vi "act_DriveQuadTalonSrx.vi"(8 "error in":errorcluster, 9 "Robot Mode":T1, 11 "QuadTalonSRXDriveRef":T2={"LeftMasterDriveRef"={"DeviceStatus"={"status"=FALSE, "code"=0, "source"=""}, "Type"=enum."PWM", "PWM"={"PWM Channel"=enum."Invalid", "DeadBand"={"Name"="", "maxPositivePwm"=0, "minPositivePwm"=0, "centerPwm"=0, "maxNegativePwm"=0, "minNegativePwm"=0, "angularRange"=0}}, "CAN"={"Device Number"=0, "SetOutput VI Ref"=variant(refnum<vi> refnum), "GetOutput VI Ref"=variant(refnum<vi> refnum), "Enable VI Ref"=variant(refnum<vi> refnum), "Disable VI Ref"=variant(refnum<vi> refnum), "Data"=variant}, "Invert"=FALSE, "DIO PWM"={"PWM \"Enable\" Channel"=enum."Invalid", "DIOChannel"=enum."Invalid", "PWM Rate"=0.0}}, "RightMasterDriveRef"={"DeviceStatus"={"status"=FALSE, "code"=0, "source"=""}, "Type"=enum."PWM", "PWM"={"PWM Channel"=enum."Invalid", "DeadBand"={"Name"="", "maxPositivePwm"=0, "minPositivePwm"=0, "centerPwm"=0, "maxNegativePwm"=0, "minNegativePwm"=0, "angularRange"=0}}, "CAN"={"Device Number"=0, "SetOutput VI Ref"=variant(refnum<vi> refnum), "GetOutput VI Ref"=variant(refnum<vi> refnum), "Enable VI Ref"=variant(refnum<vi> refnum), "Disable VI Ref"=variant(refnum<vi> refnum), "Data"=variant}, "Invert"=FALSE, "DIO PWM"={"PWM \"Enable\" Channel"=enum."Invalid", "DIOChannel"=enum."Invalid", "PWM Rate"=0.0}}}) -> (0 "error out":errorcluster)   [LabVIEW 2019, in "DriveQuadTalonSRX_Motor.lvlib"]
doc: "This VI is called for each TeleOp packet received from the DS where the robot is not disabled. It is often used to read from the joysticks and update I/O or to update setpoints for timed control loops. It should complete and return within 20 milliseconds or it may miss DS packets."
uses:
  DriveQuadTalonSRX_Motor.lvlib
  <vilib>/Rock Robotics/WPI/ThirdParty/Phoenix-LabVIEW/Motor Controller/Controls/CTRE_Phoenix_MotorControl_ControlMode.ctl
  globals_DriveQuadTalonSRX.vi
  <vilib>/Rock Robotics/SystemInterfaces/DIO/FPGA_DIOPWMChannel.ctl
  <vilib>/Rock Robotics/WPI/PWM/WPI_PWMDeadband.ctl
  <vilib>/Rock Robotics/WPI/MotorControl/WPI_MotorControlType.ctl
  <vilib>/Rock Robotics/SystemInterfaces/DIO/FPGA_DIOChannel.ctl
  <vilib>/Rock Robotics/WPI/MotorControl/WPI_MotorControlDeviceRef.ctl
  ctrlRef_DriveQuadTalon.ctl
  <vilib>/Rock Robotics/WPI/DriverStation/WPI_DriverStationRobotMode2.ctl
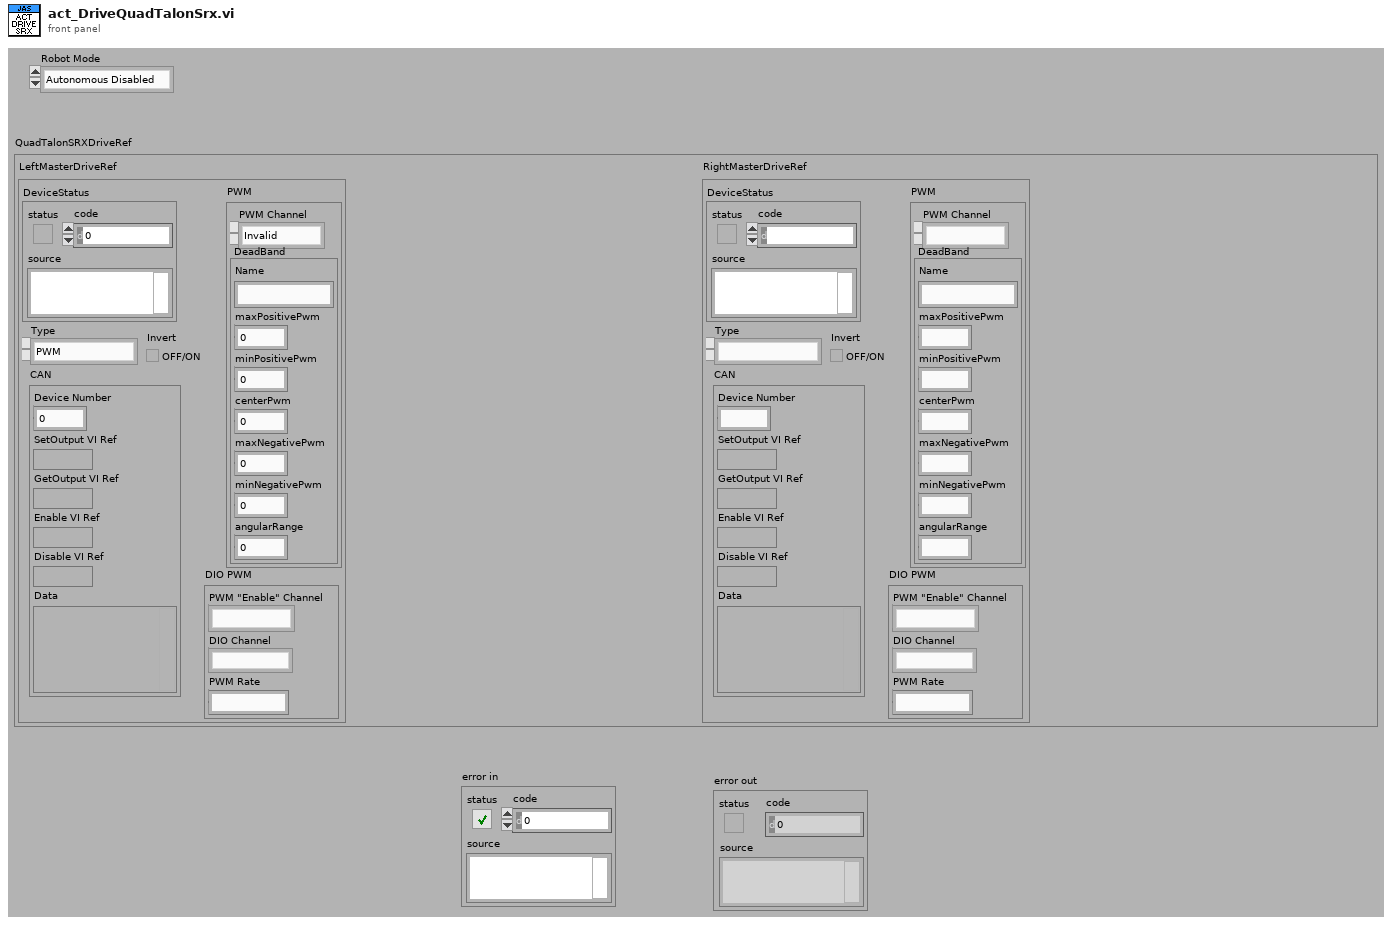
[diagram p1: front panel]
types:
  T1 = typedef "WPI_DriverStationRobotMode2.ctl" = enum16{"Autonomous Disabled", "Autonomous Enabled", "Teleop Disabled", "Teleop Enabled", "Disconnected", "Finish", "Test Disabled", "Test Enabled", "Emergency Stopped"}
  T2 = typedef "DriveQuadTalonSRX_Motor.lvlib/ctrlRef_DriveQuadTalon.ctl" = cluster{"LeftMasterDriveRef":T3, "RightMasterDriveRef":T3}
  T3 = typedef "WPI_MotorControlDeviceRef.ctl" = cluster{"DeviceStatus":errorcluster, "Type":T4, "PWM":cluster{"PWM Channel":T5, "DeadBand":T6}, "CAN":cluster{"Device Number":u8, "SetOutput VI Ref":variant, "GetOutput VI Ref":variant, "Enable VI Ref":variant, "Disable VI Ref":variant, "Data":variant}, "Invert":bool, "DIO PWM":cluster{"PWM \"Enable\" Channel":T5, "DIOChannel":T7, "PWM Rate":dbl}}
  T4 = typedef "WPI_MotorControlType.ctl" = enum16{"PWM", "CAN", "DIO PWM"}
  T5 = typedef "FPGA_DIOPWMChannel.ctl" = enum8{"PWM 0", "PWM 1", "PWM 2", "PWM 3", "PWM 4", "PWM 5", "PWM 6", "PWM 7", "PWM 8", "PWM 9", "PWM MXP 0", "PWM MXP 1", "PWM MXP 2", "PWM MXP 3", "PWM MXP 4", "PWM MXP 5", "PWM MXP 6", "PWM MXP 7", "PWM MXP 8", "PWM MXP 9", "Invalid"}
  T6 = typedef "WPI_PWMDeadband.ctl" = cluster{"Name":string, "maxPositivePwm":i32, "minPositivePwm":i32, "centerPwm":i32, "maxNegativePwm":i32, "minNegativePwm":i32, "angularRange":u16}
  T7 = typedef "FPGA_DIOChannel.ctl" = enum8{"DIO 0", "DIO 1", "DIO 2", "DIO 3", "DIO 4", "DIO 5", "DIO 6", "DIO 7", "DIO 8", "DIO 9", "DIO MXP 0", "DIO MXP 1", "DIO MXP 2", "DIO MXP 3", "DIO MXP 4", "DIO MXP 5", "DIO MXP 6", "DIO MXP 7", "DIO MXP 8", "DIO MXP 9", "DIO MXP 10", "DIO MXP 11", "DIO MXP 12", "DIO MXP 13", "DIO MXP 14", "DIO MXP 15", "SPI Port CS1", "SPI Port CS2", "SPI Port CS3", "SPI Port MISO", "SPI Port MOSI", "Invalid"}
  T8 = typedef "CTRE_Phoenix_MotorControl_ControlMode.ctl" = u16
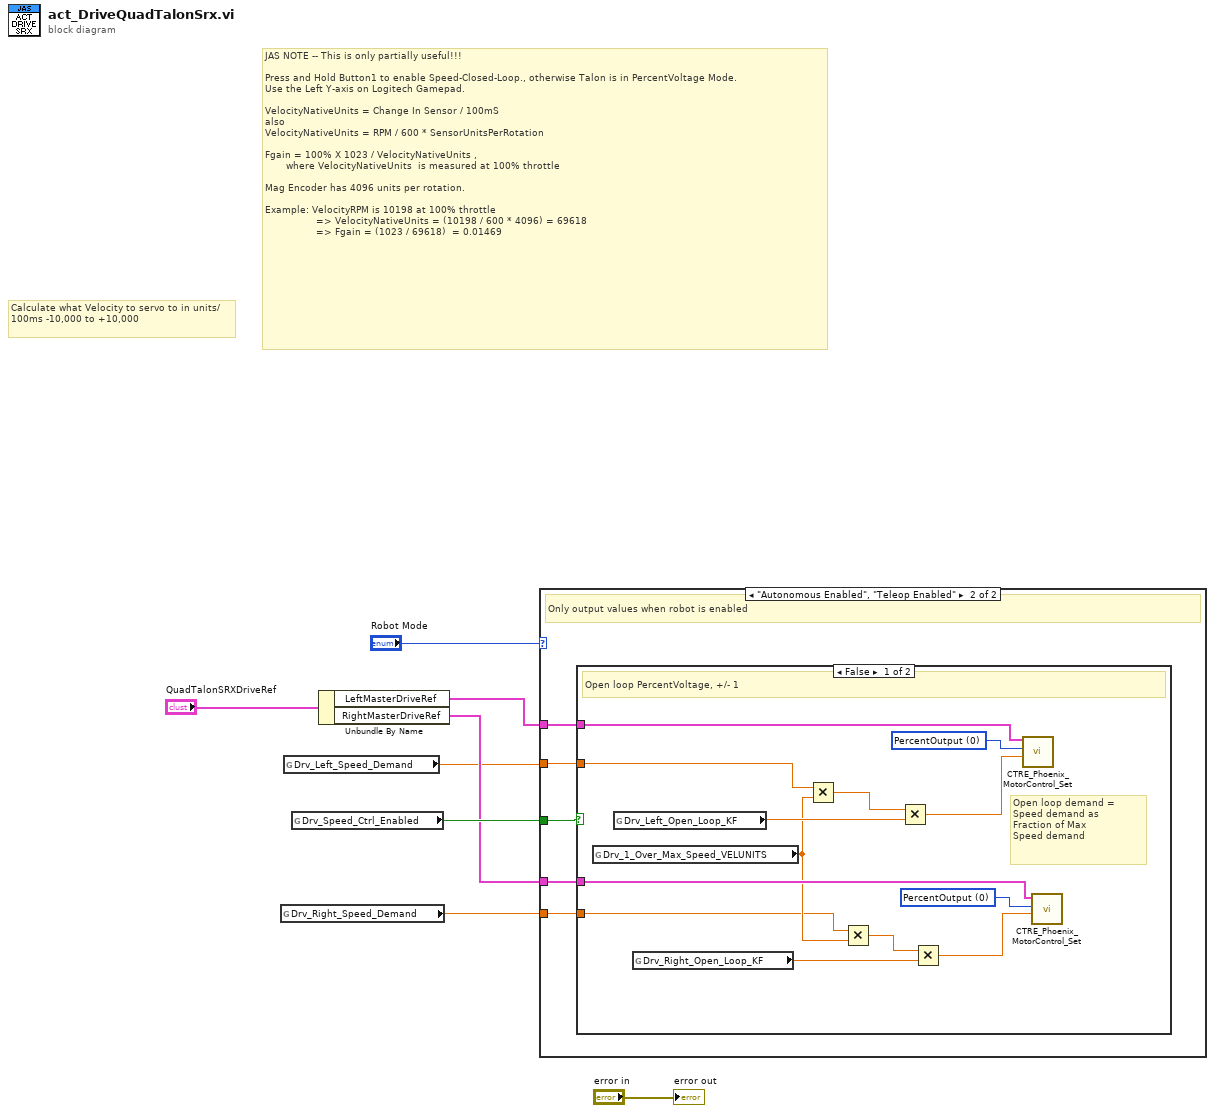
[diagram p0: block diagram]
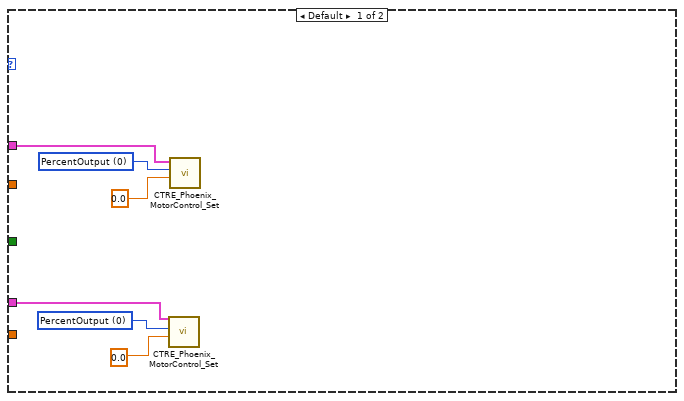
[diagram p2: hidden frame]
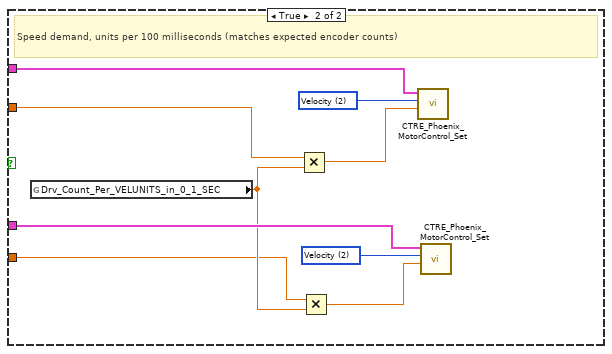
[diagram p3: hidden frame]
diagram:
  # "JAS NOTE -- This is only partially useful!!!\n\nPress and Hold Button1 to enable Speed-Closed-Loop., otherwise Talon is in PercentVoltage Mode.  \nUse the Left Y-axis on Logitech Gamepad.\n\nVelocityNativeUnits = Change In Sensor / 100mS\nalso\nVelocityNativeUnits = RPM / 600 * SensorUnitsPerRotation\n\nFgain = 100% X 1023 / VelocityNativeUnits , \n       where VelocityNativeUnits  is measured at 100% throttle\n\nMag Encoder has 4096 units per rotation.\n\nExample: VelocityRPM is 10198 at 100% throttle\n                 => VelocityNativeUnits = (10198 / 600 * 4096) = 69618\n                 => Fgain = (1023 / 69618)  = 0.01469"
  # "Calculate what Velocity to servo to in units/100ms -10,000 to +10,000"
  n1 = global read "globals_DriveQuadTalonSRX.vi" "Drv_Right_Speed_Demand"() -> (w2:dbl)
  n2 = global read "globals_DriveQuadTalonSRX.vi" "Drv_Left_Speed_Demand"() -> (w3:dbl)
  n3 = global read "globals_DriveQuadTalonSRX.vi" "Drv_Speed_Ctrl_Enabled"() -> (w7:bool)
  n4 = Unbundle By Name("QuadTalonSRXDriveRef") -> ("LeftMasterDriveRef"=w6:T3, "RightMasterDriveRef"=w5:T3)
  n5 = case shown="\"Autonomous Enabled\", \"Teleop Enabled\"" "Robot Mode" {
    tunnel: w7 -> [_ w19]
    tunnel: w6 -> [w11 w18]
    tunnel: w5 -> [w10 w17]
    tunnel: w3 -> [_ w16]
    tunnel: w2 -> [_ w15]
    frame Default {
      w13 = T8 0 items=["PercentOutput"=0, "Position"=1, "Velocity"=2, "Follower"=5, "MotionProfile"=6, "MotionMagic"=7, "MotionMagicArc"=8, "TimedPercentOutput"=9, "Disabled"=15] ("Control Mode")
      w14 = T8 0 items=["PercentOutput"=0, "Position"=1, "Velocity"=2, "Follower"=5, "MotionProfile"=6, "MotionMagic"=7, "MotionMagicArc"=8, "TimedPercentOutput"=9, "Disabled"=15] ("Control Mode")
      n6 = call <vilib>:"CTRE_Phoenix_MotorControl_Set.vi"("Output"=0.0, "Control Mode"=w13, "PhoenixMotorControlDevRef"=w10) -> ()  [unwired: 7 in, 2 out]
      n7 = call <vilib>:"CTRE_Phoenix_MotorControl_Set.vi"("Output"=0.0, "Control Mode"=w14, "PhoenixMotorControlDevRef"=w11) -> ()  [unwired: 7 in, 2 out]
    }
    frame "Autonomous Enabled", "Teleop Enabled" {
      # "Only output values when robot is enabled"
      n8 = case shown="False" w19 {
        tunnel: w18 -> [w32 w40]
        tunnel: w17 -> [w30 w38]
        tunnel: w16 -> [w24 w35]
        tunnel: w15 -> [w20 w36]
        frame False {
          w23 = T8 0 items=["PercentOutput"=0, "Position"=1, "Velocity"=2, "Follower"=5, "MotionProfile"=6, "MotionMagic"=7, "MotionMagicArc"=8, "TimedPercentOutput"=9, "Disabled"=15] ("Control Mode")
          w31 = T8 0 items=["PercentOutput"=0, "Position"=1, "Velocity"=2, "Follower"=5, "MotionProfile"=6, "MotionMagic"=7, "MotionMagicArc"=8, "TimedPercentOutput"=9, "Disabled"=15] ("Control Mode")
          # "Open loop demand = \nSpeed demand as\nFraction of Max\nSpeed demand"
          # "Open loop PercentVoltage, +/- 1"
          n9 = global read "globals_DriveQuadTalonSRX.vi" "Drv_1_Over_Max_Speed_VELUNITS"() -> (w25:dbl)
          n10 = global read "globals_DriveQuadTalonSRX.vi" "Drv_Left_Open_Loop_KF"() -> (w28:dbl)
          n11 = global read "globals_DriveQuadTalonSRX.vi" "Drv_Right_Open_Loop_KF"() -> (w29:dbl)
          n12 = Multiply(x=w24, y=w25) -> (x*y=w26:dbl)
          n13 = Multiply(x=w20, y=w25) -> (x*y=w27:dbl)
          n14 = Multiply(x=w26, y=w28) -> (x*y=w21:dbl)
          n15 = Multiply(x=w27, y=w29) -> (x*y=w22:dbl)
          n16 = call <vilib>:"CTRE_Phoenix_MotorControl_Set.vi"("Output"=w21, "Control Mode"=w31, "PhoenixMotorControlDevRef"=w32) -> ()  [unwired: 7 in, 2 out]
          n17 = call <vilib>:"CTRE_Phoenix_MotorControl_Set.vi"("Output"=w22, "Control Mode"=w23, "PhoenixMotorControlDevRef"=w30) -> ()  [unwired: 7 in, 2 out]
        }
        frame True {
          w39 = T8 2 items=["PercentOutput"=0, "Position"=1, "Velocity"=2, "Follower"=5, "MotionProfile"=6, "MotionMagic"=7, "MotionMagicArc"=8, "TimedPercentOutput"=9, "Disabled"=15] ("Control Mode")
          w41 = T8 2 items=["PercentOutput"=0, "Position"=1, "Velocity"=2, "Follower"=5, "MotionProfile"=6, "MotionMagic"=7, "MotionMagicArc"=8, "TimedPercentOutput"=9, "Disabled"=15] ("Control Mode")
          # "Speed demand, units per 100 milliseconds (matches expected encoder counts)"
          n18 = global read "globals_DriveQuadTalonSRX.vi" "Drv_Count_Per_VELUNITS_in_0_1_SEC"() -> (w37:dbl)
          n19 = Multiply(x=w35, y=w37) -> (x*y=w33:dbl)
          n20 = Multiply(x=w36, y=w37) -> (x*y=w34:dbl)
          n21 = call <vilib>:"CTRE_Phoenix_MotorControl_Set.vi"("Output"=w33, "Control Mode"=w41, "PhoenixMotorControlDevRef"=w40) -> ()  [unwired: 7 in, 2 out]
          n22 = call <vilib>:"CTRE_Phoenix_MotorControl_Set.vi"("Output"=w34, "Control Mode"=w39, "PhoenixMotorControlDevRef"=w38) -> ()  [unwired: 7 in, 2 out]
        }
      }
    }
  }
  "error out" <- "error in"
